vi "Stop Work.vi"(8 "error in (no error)":errorcluster, 9 "Reply":bool=TRUE, 10 "Reply to":refnum<class "Stop Response Msg.lvclass">, 11 "Spectrum Recorder in":refnum<class "Spectrum Recorder too.lvclass">) -> (0 "error out":errorcluster, 3 "Spectrum Recorder out":refnum<class "Spectrum Recorder too.lvclass">)   [LabVIEW 2016, in "Spectrum Recorder too.lvclass"]
uses:
  Spectrum Recorder too.lvclass
  Controllers/Process Controller Messages/Stop Response Msg/Stop Response Msg.lvclass
  Spectrum Recorder too.lvclass/Spectrum Recorder too.ctl
  Read RP transceiver.vi
  Write RP transceiver.vi
  NHMFL_Core/Libraries/Red Pitaya/RP Core/RP Transceiver/RP Transceiver.lvclass
  Instrument Actor/Instrument Actor.lvclass
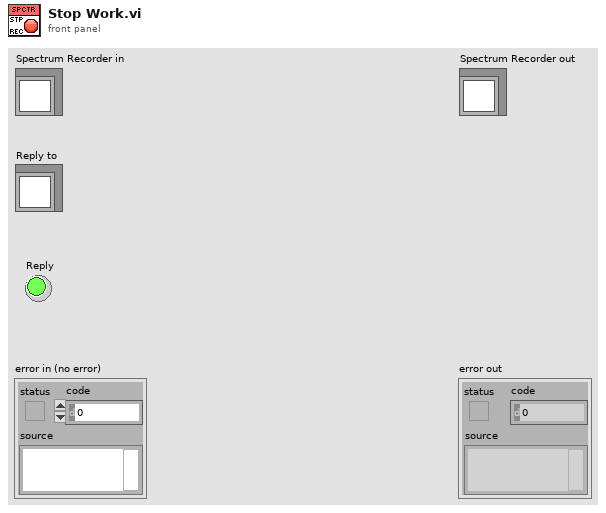
[diagram p1: front panel]
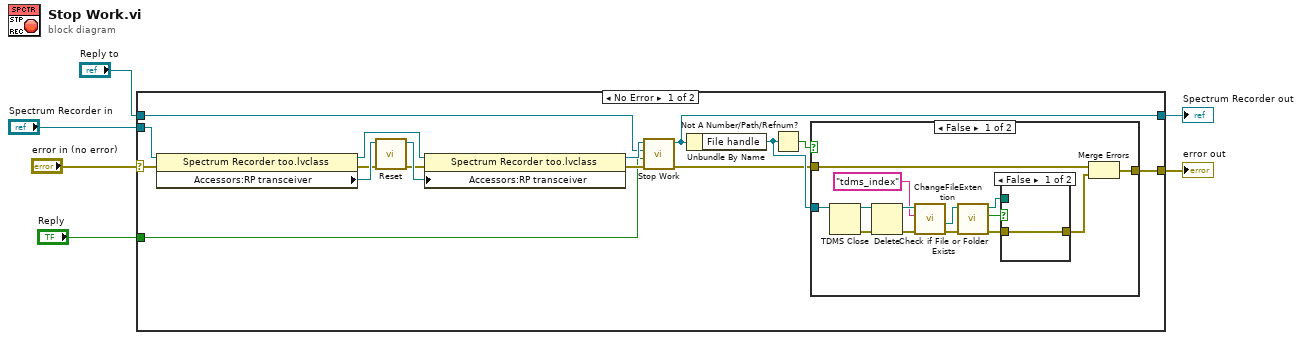
[diagram p0: block diagram]
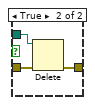
[diagram p2: hidden frame]
diagram:
  n1 = case shown="No Error" "error in (no error)" {
    selector: "error in (no error)" -> [w20 w43]
    tunnel: [w9 w43] -> w5
    tunnel: [w11 w42] -> w3
    tunnel: "Spectrum Recorder in" -> [w17 w42]
    tunnel: "Reply to" -> [w8 _]
    tunnel: "Reply" -> [w7 _]
    frame No Error {
      n2 = property class="Spectrum Recorder too.lvclass"(reference=w17, error in=w20) -> (reference out=w12:refnum<class "Spectrum Recorder too.lvclass">, error out=w13:errorcluster, "Accessors:RP transceiver"=w19:refnum<class "RP Transceiver.lvclass">)
      n3 = call-dynamic "Reset.vi"("error in (no error)"=w13, "RP Instrument in"=w19) -> ("error out"=w14:errorcluster, "RP Instrument out"=w18:refnum<class "RP Transceiver.lvclass">)  [unwired: 8 in]
      n4 = property class="Spectrum Recorder too.lvclass"(reference=w12, error in=w14, "Accessors:RP transceiver"=w18) -> (reference out=w16:refnum<class "Spectrum Recorder too.lvclass">, error out=w15:errorcluster)
      n5 = call-parent "Stop Work.vi"("error in (no error)"=w15, "Reply"=w7, "Reply to"=w8, "Measure Object in"=w16) -> ("error out"=w10:errorcluster, "Measure Object out"=w11:refnum<class "Spectrum Recorder too.lvclass">)  [unwired: 6 in]
      n6 = Unbundle By Name(w11) -> ("File handle"=w21:refnum<k34>)
      n7 = Not A Number/Path/Refnum?(number/path/refnum=w21) -> (NaN/Path/Refnum?=w22:bool)
      n8 = case shown="False" w22 {
        tunnel: w21 -> [w36 _]
        tunnel: w10 -> [w28 w41]
        tunnel: [w26 w41] -> w9
        frame False {
          n9 = TDMS Close(11:w36) -> (0:w34:errorcluster, 3:w35:path)  [unwired: 1 in]
          n10 = Delete(path (use dialog)=w35, error in=w34) -> (deleted path=w33:path, error out=w25:errorcluster)  [unwired: 3 in, 1 out]
          n11 = call "ChangeFileExtention.vi"("Error In"=w25, "New extension"="tdms_index" ("New Extention"), "File Path"=w33) -> ("Error Out"=w24:errorcluster, "Path with new extension"=w23:path)  [unwired: 3 in, 4 out]
          n12 = call <vilib>:"Check if File or Folder Exists.vi"("error in (no error)"=w24, "path"=w23) -> ("error out"=w30:errorcluster, "file or folder exists?"=w31:bool, "dup path"=w29:path)  [unwired: 7 in]
          n13 = case shown="False" w31 {
            tunnel: w30 -> [w37 w40]
            tunnel: w29 -> [_ w39]
            tunnel: [w37 w38] -> w27
            frame False {
            }
            frame True {
              n14 = Delete(path (use dialog)=w39, error in=w40) -> (error out=w38:errorcluster)  [unwired: 3 in, 2 out]
            }
          }
          n15 = Merge Errors(w28, w27) -> (w26:errorcluster)
        }
        frame True {
        }
      }
    }
    frame Error {
    }
  }
  "error out" <- w5
  "Spectrum Recorder out" <- w3
